vi "Config Panel.vi"(8 "error in (no error)":errorcluster, 11 "AD4212C in":refnum<class "AD4212C.lvclass">) -> (0 "error out":errorcluster, 3 "AD4212C out":refnum<class "AD4212C.lvclass">)   [LabVIEW 2014, in "AD4212C.lvlib" / "AD4212C.lvclass"]
doc: "Calibra la balanza y configura el puerto COM. Llama a los VIs correspondientes que ejecutan dichas tareas."
uses:
  AD4212CClass/AD4212C.lvclass
  AD4212CClass/AD4212C.lvclass/AD4212C.ctl
  API/AD4212C Lib.lvlib
panel:
  in  "Config":bool
  in  "Calibration":bool
  # "CONFIGURACIÓN"
  # "(Antes de Calibrar siempre configurar el puerto)"
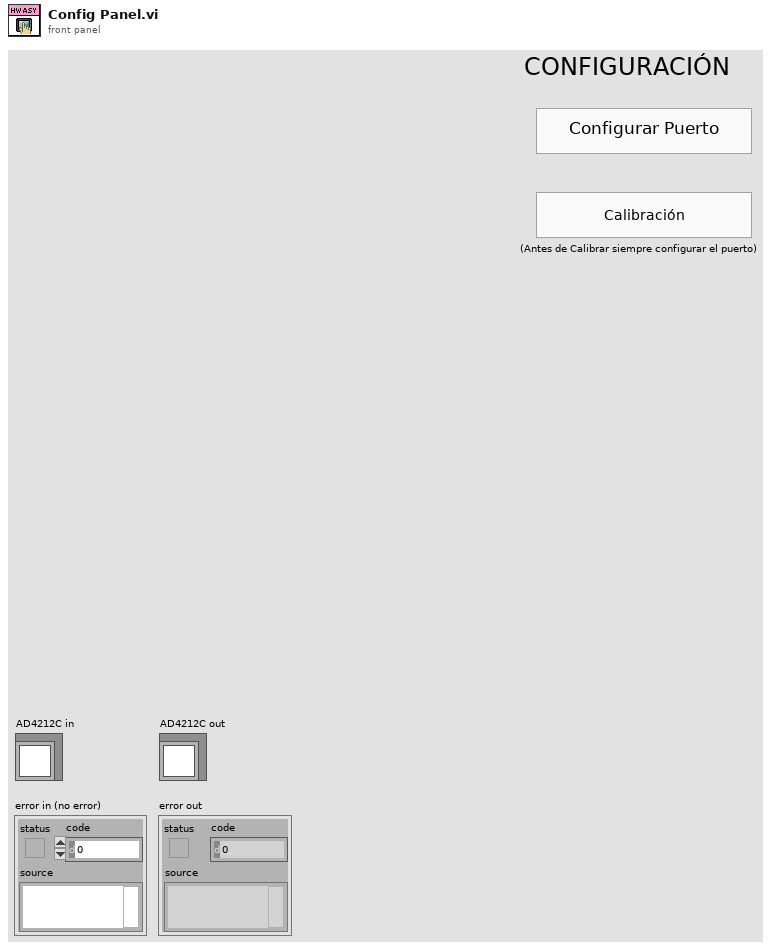
[diagram p1: front panel]
types:
  T1 = typedef "AD4212C Lib.lvlib/Connection Data.ctl" = cluster{"Conection Data":refnum<visa-resource-name>}
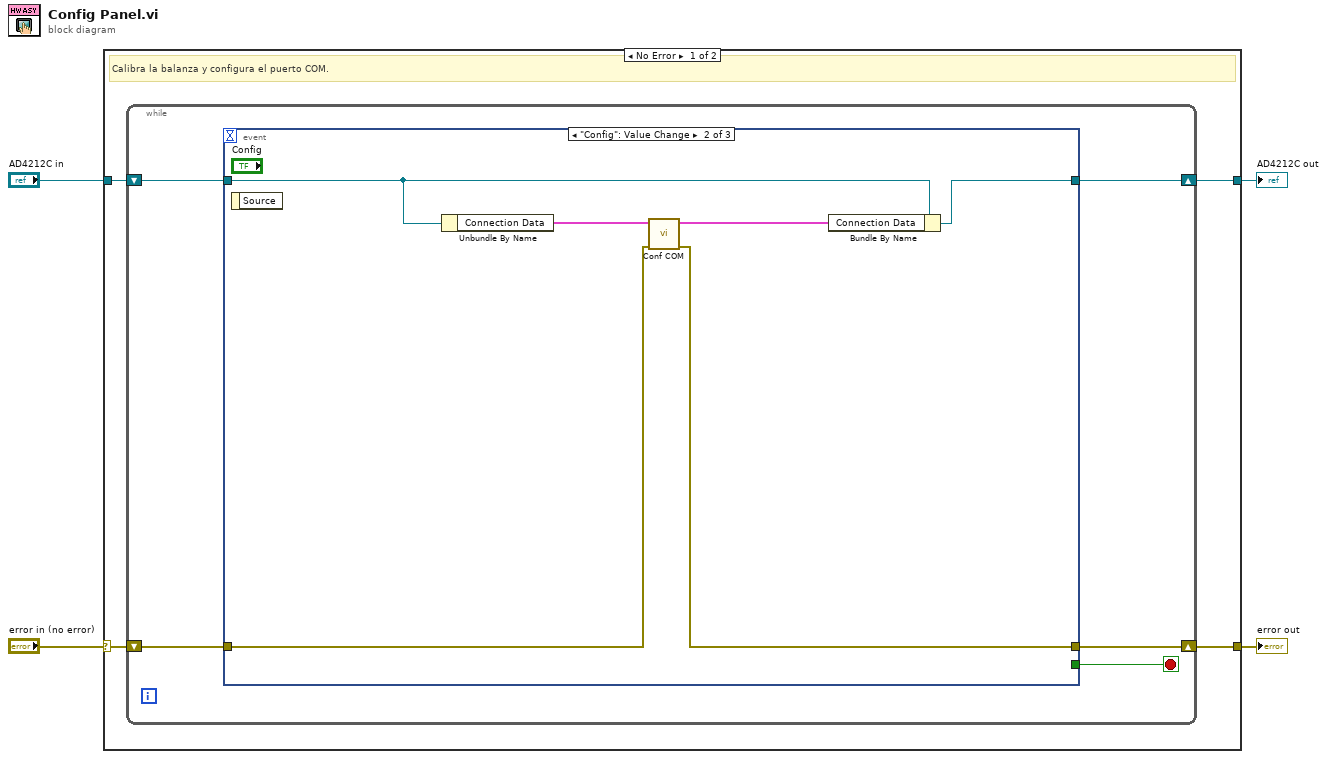
[diagram p0: block diagram]
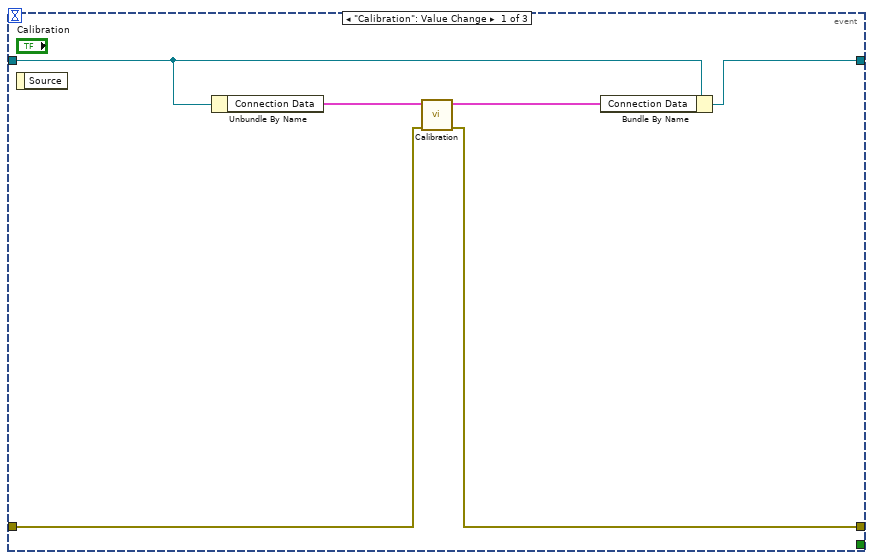
[diagram p2: hidden frame]
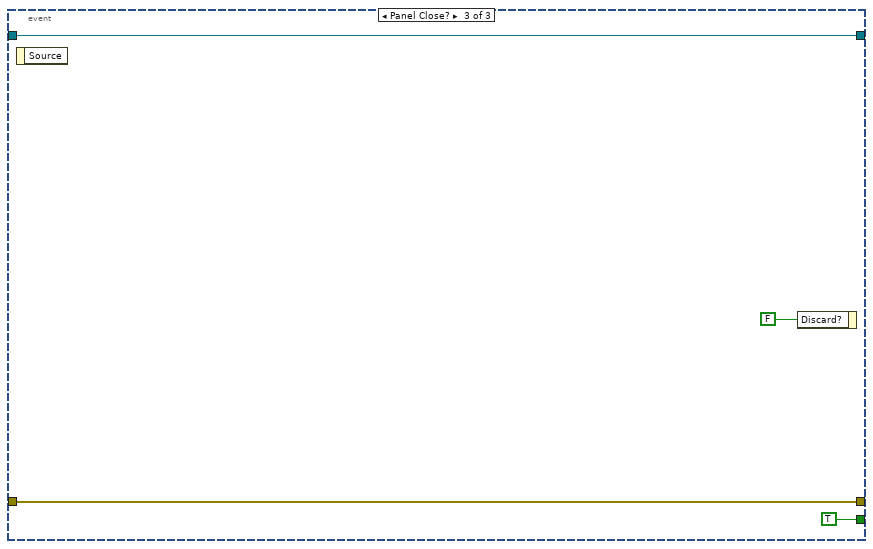
[diagram p3: hidden frame]
diagram:
  n1 = case shown="No Error" "error in (no error)" {
    selector: "error in (no error)" -> [w5 w31]
    tunnel: [w6 w31] -> w3
    tunnel: [w8 w30] -> w1
    tunnel: "AD4212C in" -> [w7 w30]
    frame No Error {
      # "Calibra la balanza y configura el puerto COM."
      n2 = while {
        shift-right: [w13] -> w8
        shift-left: w7 -> [w12]
        shift-right: [w11] -> w6
        shift-left: w5 -> [w10]
        stop <- w9 stop-if-true
        n3 = event shown="[1] \"Config\": Value Change" {
          selector: _ -> [_ _ _]
          dyn-events: _ -> [_ _ _]
          timeout: _ -> [_ _ _]
          tunnel: [w19 w25 w26] -> w13
          tunnel: w12 -> [w18 w24 w26]
          tunnel: [w14 w20 w27] -> w11
          tunnel: w10 -> [w15 w21 w27]
          tunnel: [_ _ TRUE ("Discard?")] -> w9
          event "Calibration": Value Change {
            n4 = event-data() -> ()  [unwired: 1 in, 1 out]
            n5 = Unbundle By Name(w18) -> ("Connection Data"=w17:T1)
            n6 = call "Calibration.vi"("error in (no error)"=w15, "VISA resource name In"=w17) -> ("error out"=w14:errorcluster, "VISA resource name Out"=w16:T1)  [unwired: 8 in]
            n7 = Bundle By Name(cluster=w18, "Connection Data"=w16) -> (w19:refnum<class "AD4212C.lvclass">)
          }
          event "Config": Value Change {
            n8 = event-data() -> ()  [unwired: 1 in, 1 out]
            n9 = Unbundle By Name(w24) -> ("Connection Data"=w23:T1)
            n10 = call "Conf COM.vi"("error in (no error)"=w21, "Conection Data"=w23) -> ("error out (no error)"=w20:errorcluster, "Conection Data 2"=w22:T1)  [unwired: 8 in]
            n11 = Bundle By Name(cluster=w24, "Connection Data"=w22) -> (w25:refnum<class "AD4212C.lvclass">)
          }
          event Panel Close? {
            n12 = event-data() -> ()  [unwired: 1 in, 1 out]
            n13 = event-data("Discard?"=FALSE) -> ()  [unwired: 1 in, 1 out]
          }
        }
      }
    }
    frame Error {
    }
  }
  "error out" <- w3
  "AD4212C out" <- w1
